vi "XNET Flush.vi"(0 "session in":refnum<k21>, 11 "error in (no error)":errorcluster) -> (4 "session out":refnum<k21>, 15 "error out":errorcluster)   [LabVIEW 2018]
doc: "Flush all queues for this session. This discards the values in those queues. \n\nWith the exception of single-point modes, all sessions use queues to store frames. For input modes, the queues store frame values (or corresponding signal values) that have been received, but not obtained by calling the XNET Read VI. For output sessions, the queues store frame values provided to the XNET Write VI, but not transmitted successfully.\n\nThe XNET Start VI and XNET Stop VI have no effect on these queues. Use this XNET Flush VI to discard all values in the session's queues.\n\nFor example, if you call the XNET Write VI to write three frames, then immediately call the XNET Stop VI, then call the XNET Start VI a few seconds later, the three frames transmit. If you call the XNET Flush VI between the XNET Stop VI and XNET Start VI, no frames transmit."
uses:
  nixlvapi.dll
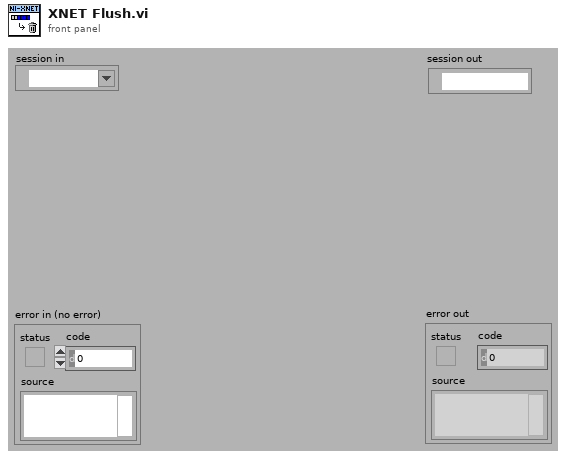
[diagram p1: front panel]
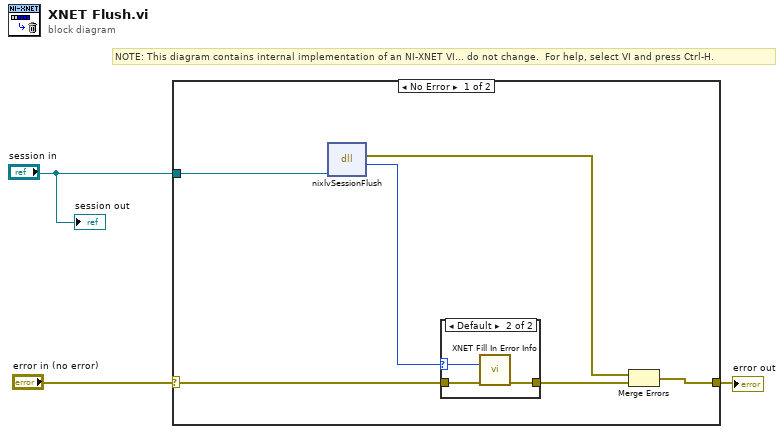
[diagram p0: block diagram]
diagram:
  # "NOTE: This diagram contains internal implementation of an NI-XNET VI... do not change.  For help, select VI and press Ctrl-H."
  n1 = case shown="No Error" "error in (no error)" {
    selector: "error in (no error)" -> [w8 w14]
    tunnel: "session in" -> [w9 _]
    tunnel: [w5 w14] -> w3
    frame No Error {
      # "NOTE: This diagram contains internal implementation of an NI-XNET VI... do not change.  For help, select VI and press Ctrl-H."
      n2 = dll-call lib="nixlvapi.*" fn="nixlvSessionFlush" ("nilvxaiu.dll:lvxenSessionClear")("reference"=w9) -> (error out=w4:errorcluster, "return type"=w6:i32)  [unwired: 3 in, 2 out]
      n3 = case shown="Default" w6 {
        selector: w6 -> [_ w11]
        tunnel: w8 -> [w10 w12]
        tunnel: [w10 w13] -> w7
        frame 0 {
        }
        frame Default {
          n4 = call "XNET Fill In Error Info.vi"("status code"=w11, "error in"=w12) -> ("error out"=w13:errorcluster)  [unwired: 13 out]
        }
      }
      n5 = Merge Errors(w4, w7) -> (w5:errorcluster)
    }
    frame Error {
    }
  }
  "error out" <- w3
  "session out" <- "session in"
